vi "Delete Record Query SQLServer.vi"(7 "Where":string, 8 "error in (no error)":errorcluster, 10 "Table":string, 11 "ADODB._Connection":refnum<k7>) -> (0 "error out":errorcluster, 2 "Records Affected":i32, 3 "ADODB._Connection 2":refnum<k7>)   [LabVIEW 2017]
panel:
  out "Query":string
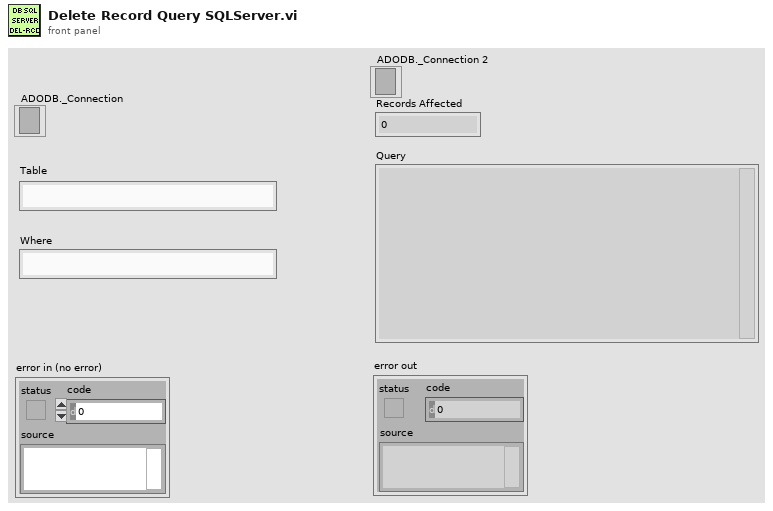
[diagram p1: front panel]
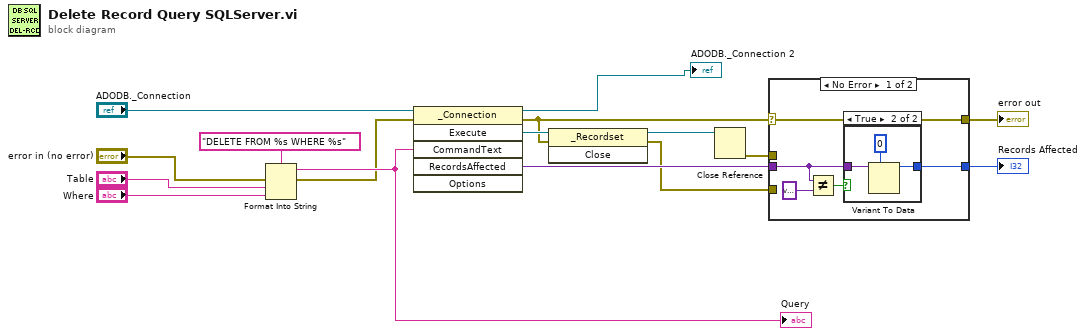
[diagram p0: block diagram]
diagram:
  n1 = Format Into String(format string="DELETE FROM %s WHERE %s", error in="error in (no error)", "Table", "Where") -> (resulting string=w13:string, error out=w9:errorcluster)  [unwired: 1 in]
  "Query" <- w13
  n2 = invoke class="_Connection" method="Execute"(reference="ADODB._Connection", error in=w9, "CommandText"=w13) -> (reference out=→"ADODB._Connection 2":refnum<k7>, error out=w5:errorcluster, "Execute"=w6:refnum<k7>, "RecordsAffected"=w11:variant)  [unwired: 3 in, 2 out]
  n3 = invoke class="_Recordset" method="Close"(reference=w6, error in=w5) -> (reference out=w4:refnum<k7>, error out=w2:errorcluster)  [unwired: 1 in, 1 out]
  n4 = Close Reference(reference=w4) -> (error out=w3:errorcluster)  [unwired: 1 in]
  n5 = case shown="No Error" w5 {
    selector: w5 -> [w17 w25]
    tunnel: [w17 w25] -> w12
    tunnel: w11 -> [w20 _]
    tunnel: [w21 _] -> w10
    tunnel: w3 -> [_ _]
    tunnel: w2 -> [_ _]
    frame No Error {
      n6 = Not Equal?(x=w20, y=variant) -> (x != y?=w18:bool)
      n7 = case shown="True" w18 {
        tunnel: [_ w23] -> w21
        tunnel: w20 -> [_ w22]
        frame False {
        }
        frame True {
          n8 = Variant To Data(type=0, Variant=w22) -> (data=w23:i32)  [unwired: 1 in, 1 out]
        }
      }
    }
    frame Error {
    }
  }
  "error out" <- w12
  "Records Affected" <- w10
